vi "Tile Windows.vi"(7 "Tile Direction":T1 items=["Horizontal", "Vertical"], 8 "error in (no error)":errorcluster, 9 "ChildHwnd[]":u32[](array[numeric]), 10 "Child Count":i32, 11 "Parent Hwnd":i32) -> (0 "error out":errorcluster)   [LabVIEW 2019, in "LV MDI.lvclass"]
doc: "Tile child windows within the parent window."
uses:
  LV MDI.lvclass
  Typedef/Tile Direction.ctl
  user32.dll
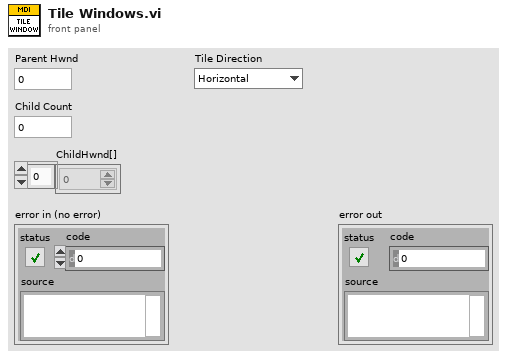
[diagram p1: front panel]
types:
  T1 = typedef "LV MDI.lvclass/Tile Direction.ctl" = u16
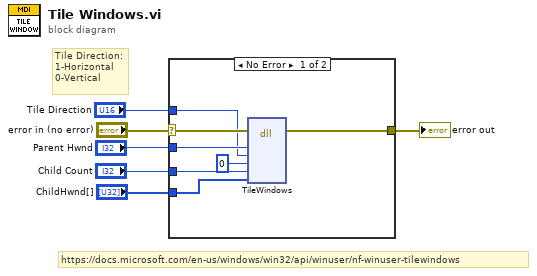
[diagram p0: block diagram]
diagram:
  # "https://docs.microsoft.com/en-us/windows/win32/api/winuser/nf-winuser-tilewindows"
  # "Tile Direction:\n1-Horizontal\n0-Vertical"
  n1 = case shown="No Error" "error in (no error)" {
    selector: "error in (no error)" -> [w12 w14]
    tunnel: [w13 w14] -> w6
    tunnel: "Child Count" -> [w11 _]
    tunnel: "Parent Hwnd" -> [w10 _]
    tunnel: "Tile Direction" -> [w9 _]
    tunnel: "ChildHwnd[]" -> [w7 _]
    frame No Error {
      n2 = dll-call lib="user32.dll" fn="TileWindows"(error in=w12, "hwndParent"=w10, "wHow"=w9, "lpRect"=0 ("wHow"), "cKids"=w11, "lpKids"=w7) -> (error out=w13:errorcluster)  [unwired: 8 in, 1 out]
    }
    frame Error {
    }
  }
  "error out" <- w6
